vi "encoder_sample.vi"   [LabVIEW 2017]
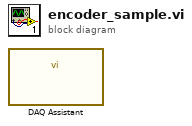
[diagram p0: block diagram]
diagram:
  n1 = call "DAQ Assistant"() -> ()  [unwired: 12 in]
